vi "MicroStageSetRelativePosition.vi"(7 "error in (no error)":errorcluster, 8 "Move size (µm)":dbl=50.0 format="%.3f", 9 "Direction":bool, 10 "Config In":T1 {"Hardware Configuration"."Lasers Configuration"."SettingValues"."785 Power" format="%.1f"; "Hardware Configuration"."Lasers Configuration"."SettingValues"."647 Power" format="%.1f"; "Hardware Configuration"."Lasers Configuration"."SettingValues"."561 Power" format="%.1f"}) -> (0 "error out":errorcluster, 3 "Config Out":T1 {"Hardware Configuration"."Lasers Configuration"."SettingValues"."785 Power" format="%.1f"; "Hardware Configuration"."Lasers Configuration"."SettingValues"."647 Power" format="%.1f"; "Hardware Configuration"."Lasers Configuration"."SettingValues"."561 Power" format="%.1f"})   [LabVIEW 2019]
doc: "Generates sample waveforms according to the signal type in the HW Config input."
uses:
  Settings/System Running Settings.ctl
  Support/Hardware Configuration.ctl
  Support/Camera Configuration.ctl
  C:/RM21-MMicrosopeSource/HardwareAdapter/Camera/Dependencies/PVCamNET.dll
  Camera/Dependencies/PVCamNET.dll
  <vilib>/vision/Image Controls.llb/IMAQ Image.ctl
  C:/RM21-MMicrosopeSource/HardwareAdapter/Lasers/Dependencies/Oxxius_Boxx.dll
  Lasers/Dependencies/Oxxius_Boxx.dll
  Logging/Logging Configuration.ctl
  Controls/DeviceStatusCtl.ctl
  Controls/CallBack Refs.ctl
  Dependencies/MicroDrive.dll
  Logging/Logging.lvlib
  Settings/Settings.lvlib
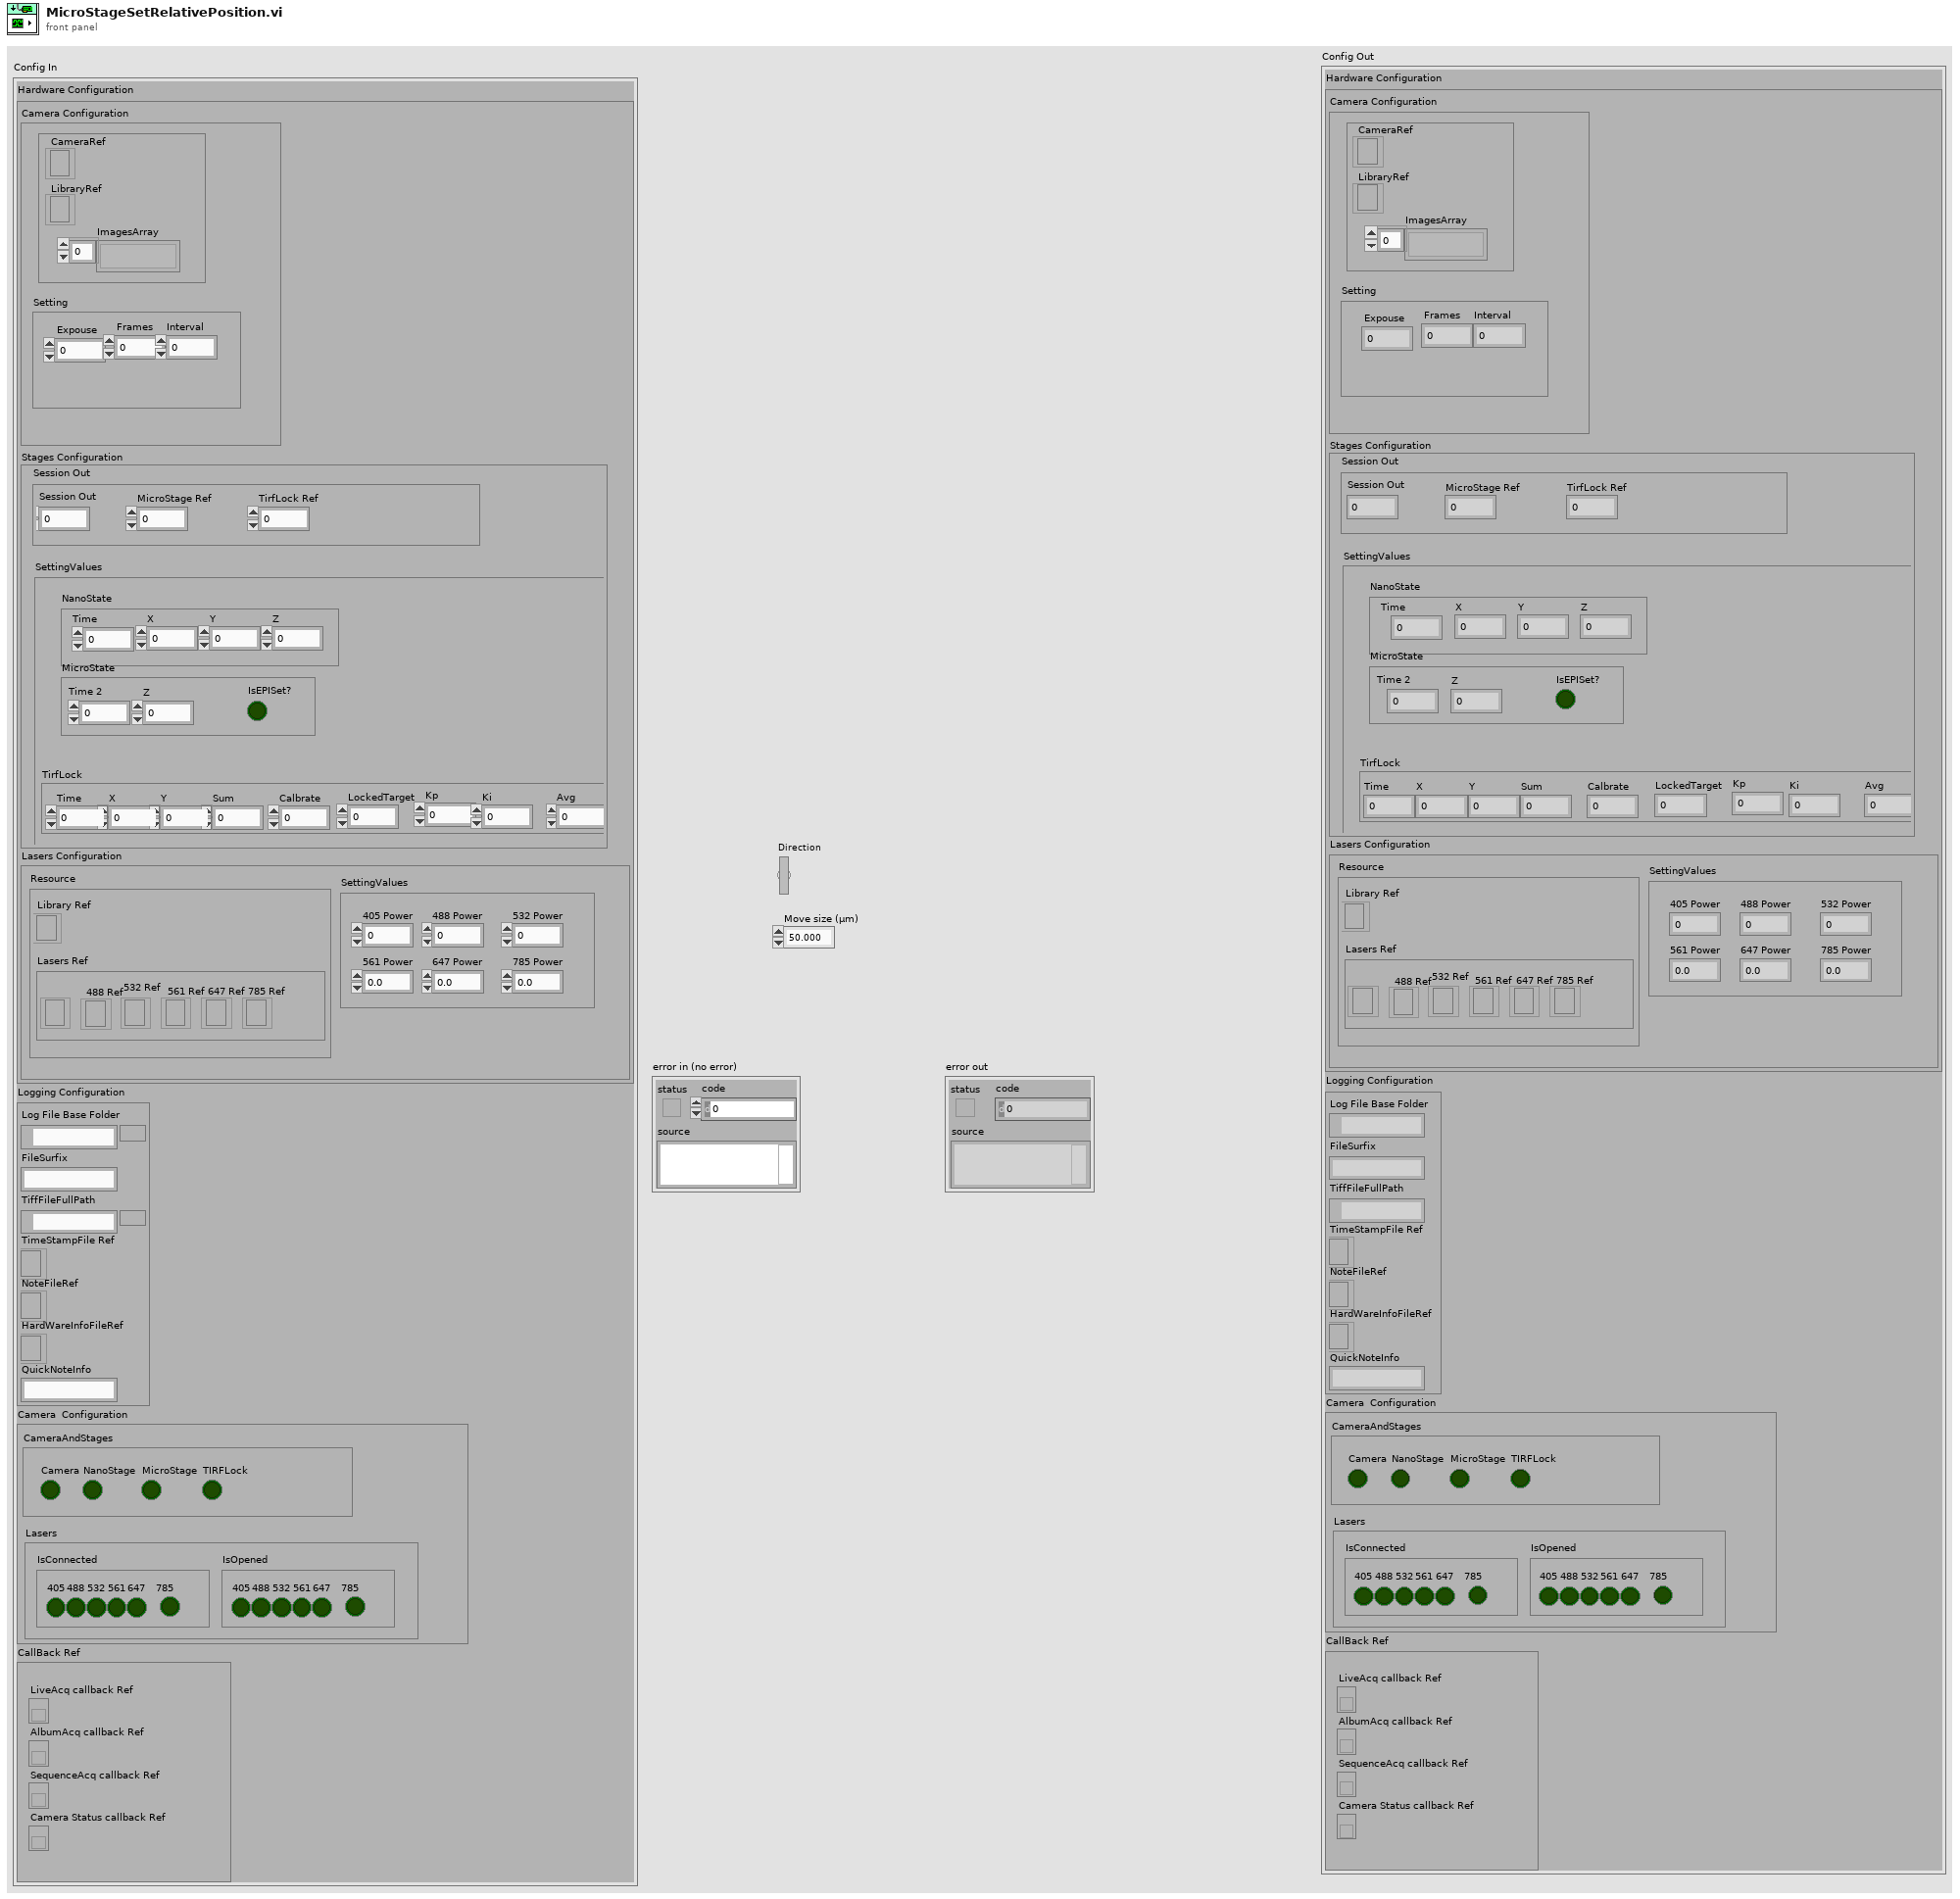
[diagram p1: front panel]
types:
  T1 = typedef "Settings.lvlib/System Running Settings.ctl" = cluster{"Hardware Configuration":T2, "Logging Configuration":T5, "HardWare Status":cluster{"CameraAndStages":T6, "Lasers":cluster{"IsConnected":cluster{"405":bool, "488":bool, "532":bool, "561":bool, "647":bool, "785":bool}, "IsOpened":cluster{"405":bool, "488":bool, "532":bool, "561":bool, "647":bool, "785":bool}}}, "CallBack Ref":T7}
  T2 = typedef "Hardware Configuration.ctl" = cluster{"Camera Configuration":T3, "Stages Configuration":cluster{"Resource":cluster{"NanoStage Ref":i32, "MicroStage Ref":i32, "TirfLock Ref":i32}, "SettingValues":cluster{"NanoState":cluster{"Time":dbl, "X":dbl, "Y":dbl, "Z":dbl}, "MicroState":cluster{"Time 2":dbl, "Z":dbl, "IsEPISet?":bool}, "TirfLock":cluster{"Time":dbl, "X":dbl, "Y":dbl, "Sum":dbl, "Calbrate":dbl, "LockedTarget":dbl, "Kp":dbl, "Ki":dbl, "Avg":dbl}}}, "Lasers Configuration":cluster{"SettingValues":cluster{"405 Power":sgl, "488 Power":sgl, "532 Power":sgl, "561 Power":sgl, "647 Power":sgl, "785 Power":sgl}, "Resource":cluster{"Library Ref":refnum<k24>, "Lasers Ref":cluster{"405 Ref":refnum<k24>, "488 Ref":refnum<k24>, "532 Ref":refnum<k24>, "561 Ref":refnum<k24>, "647 Ref":refnum<k24>, "785 Ref":refnum<k24>}}}}
  T3 = typedef "Camera Configuration.ctl" = cluster{"Setting":cluster{"Expouse":dbl, "Frames":dbl, "Interval":dbl}, "Resource":cluster{"CameraRef":refnum<k24>, "LibraryRef":refnum<k24>, "ImagesArray":T4[]}}
  T4 = typedef "IMAQ Image.ctl" = refnum<image>
  T5 = typedef "Logging.lvlib/Logging Configuration.ctl" = cluster{"Log File Base Folder":path, "FileSurfix":string, "TiffFileFullPath":path, "TimeStampFile Ref":refnum<file>, "NoteFileRef":refnum<file>, "HardWareInfoFileRef":refnum<file>, "QuickNoteInfo":string}
  T6 = typedef "DeviceStatusCtl.ctl" = cluster{"Camera":bool, "NanoStage":bool, "MicroStage":bool, "TIRFLock":bool}
  T7 = typedef "CallBack Refs.ctl" = cluster{"LiveAcq callback Ref":refnum<k27>, "AlbumAcq callback Ref":refnum<k27>, "SequenceAcq callback Ref":refnum<k27>, "Camera Status callback Ref":refnum<k27>}
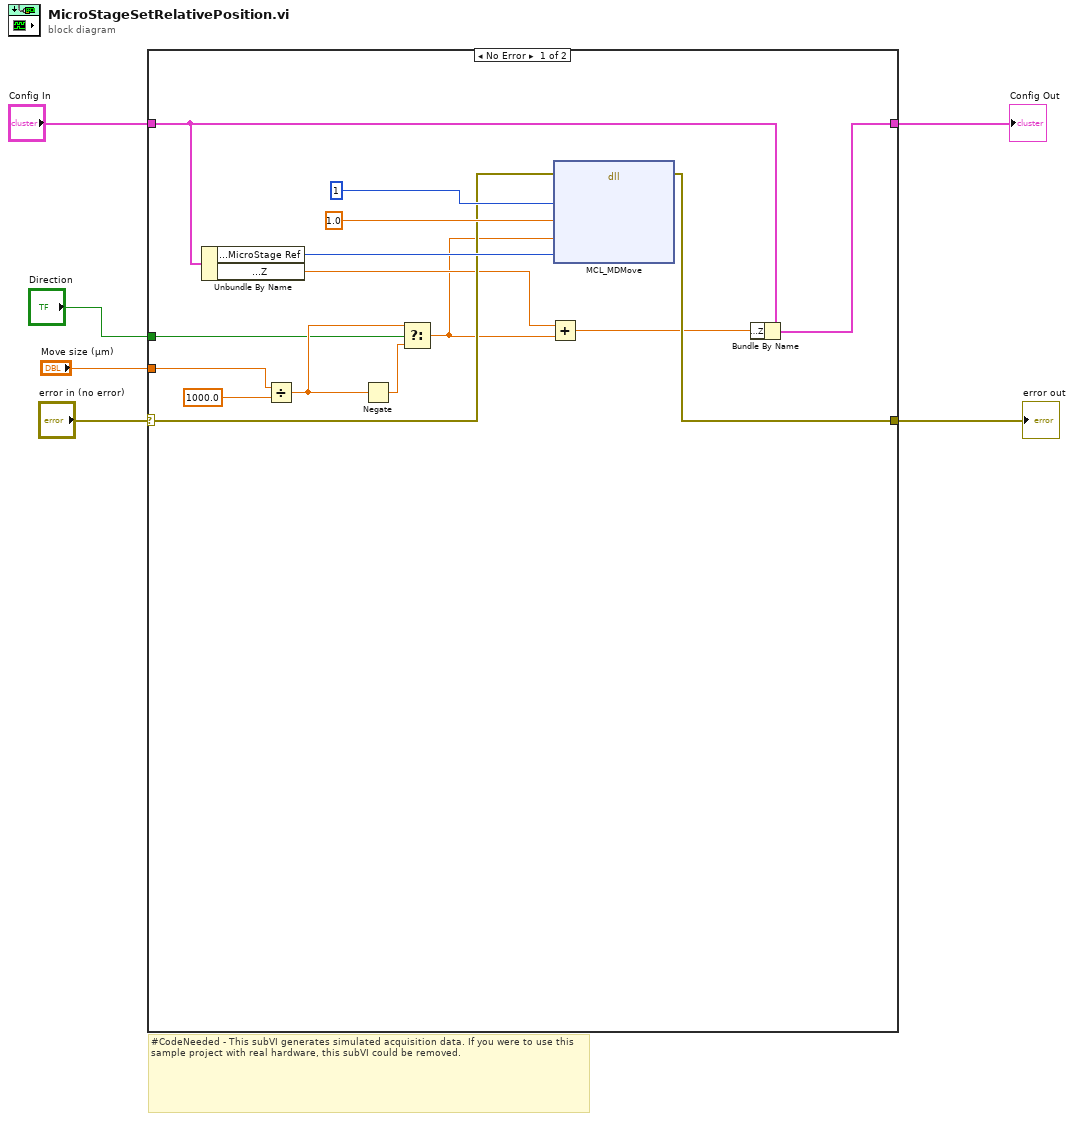
[diagram p0: block diagram]
diagram:
  # "#CodeNeeded - This subVI generates simulated acquisition data. If you were to use this sample project with real hardware, this subVI could be removed."
  n1 = case shown="No Error" "error in (no error)" {
    selector: "error in (no error)" -> [w13 w23]
    tunnel: [w12 w23] -> w5
    tunnel: "Config In" -> [w9 w22]
    tunnel: [w8 w22] -> w3
    tunnel: "Direction" -> [w14 _]
    tunnel: "Move size (µm)" -> [w15 _]
    frame No Error {
      n2 = Unbundle By Name(w9) -> ("Hardware Configuration.Stages Configuration.Resource.MicroStage Ref"=w21:i32, "Hardware Configuration.Stages Configuration.SettingValues.MicroState.Z"=w11:dbl)
      n3 = Divide(x=w15, y=1000.0) -> (x/y=w16:dbl)
      n4 = Negate(x=w16) -> (-x=w17:dbl)
      n5 = Select(t=w16, s=w14, f=w17) -> (s? t:f=w10:dbl)
      n6 = Add(x=w11, y=w10) -> (x+y=w7:dbl)
      n7 = dll-call lib="C:/RM21-MMicrosopeSource/HardwareAdapter/Stages/Dependencies/MicroDrive.dll" fn="MCL_MDMove"(error in=w13, "axis"=1, "velocity"=1.0, "distance"=w10, "handle"=w21) -> (error out=w12:errorcluster)  [unwired: 5 in, 3 out]
      n8 = Bundle By Name(cluster=w9, "Hardware Configuration.Stages Configuration.SettingValues.MicroState.Z"=w7) -> (w8:T1)
    }
    frame Error {
    }
  }
  "error out" <- w5
  "Config Out" <- w3
